vi "temp.vi"() -> ()   [LabVIEW 2017]
uses:
  Controller/Controls/UI CMD.ctl
  Controller/Controls/Controller CMD.ctl
  Error Handler/Controls/Error Data.ctl
  Configuration/Controls/Config CMD.ctl
panel:
  in  "Error UE":refnum<user-event>
  in  "Config":refnum<queue>
  in  "Error":refnum<queue>
  in  "CNTRLR":refnum<queue>
  in  "UI":refnum<queue>
  in  "Stop DVR":refnum<data-value>
  in  "Stop UE":refnum<user-event>
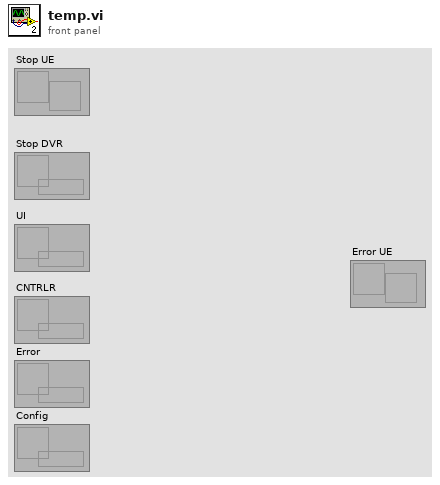
[diagram p1: front panel]
types:
  T1 = typedef "Error Data.ctl" = cluster{"Type":enum16{"Console Error", "Sensor Interface IO Error", "Process Step Error"}, "Data":variant}
  T2 = typedef "Config CMD.ctl" = cluster{"CMD":enum16{"Idle", "Read", "Search", "Update", "Stop"}, "Data":variant}
  T3 = typedef "Controller CMD.ctl" = cluster{"Command":enum16{"Init", "Terminate"}, "Data":variant}
  T4 = typedef "UI CMD.ctl" = cluster{"Command":enum16{"Idle"}, "Data":variant}
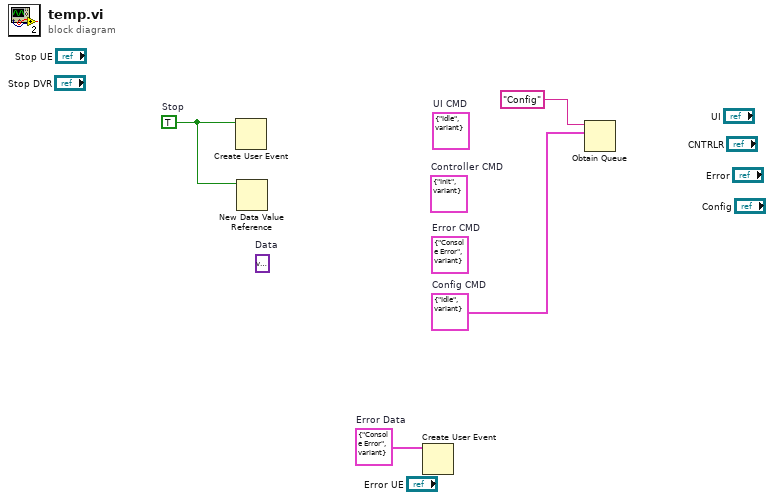
[diagram p0: block diagram]
diagram:
  w1 = T1 {"Type"=enum."Console Error", "Data"=variant}  # Error Data
  (unwired) T1 {"Type"=enum."Console Error", "Data"=variant}  # Error CMD
  w2 = T2 {"CMD"=enum."Idle", "Data"=variant}  # Config CMD
  (unwired) T3 {"Command"=enum."Init", "Data"=variant}  # Controller CMD
  (unwired) T4 {"Command"=enum."Idle", "Data"=variant}  # UI CMD
  (unwired) variant  # Data
  w4 = TRUE  # Stop
  n1 = Create User Event(user event datatype=w4) -> ()  [unwired: 1 in, 2 out]
  n2 = New Data Value Reference(data value=w4) -> ()  [unwired: 1 in, 2 out]
  n3 = Create User Event(user event datatype=w1) -> ()  [unwired: 1 in, 2 out]
  n4 = Obtain Queue(name (unnamed)="Config", element data type=w2) -> ()  [unwired: 3 in, 3 out]
